vi "DequeueCmd.vi"(8 "error in (no error)":errorcluster, 11 "queue of text strings":refnum<queue>) -> (0 "error out":errorcluster, 1 "arguments":string[](array[string]), 2 "command":string="Default", 3 "queue (dup)":refnum<queue>)   [LabVIEW 2010]
doc: "This VI serves to dequeue a command from the string queue provided to the input. The queue sorts the command from the command line arguements, which can be included after the command. The arguements are separated by a colon (:) and will be output as a string array. The VI will also handle any error that exists in the error cluster by setting the command = Error with the error code and error string message as arguments.\n\nInputs:\nqueue - input queue (string)\nerror in - error input cluster\n\nOutputs:\ncommand - main state in the queue; this is used as the current state to be used by the case structure\narguments - command line arguments that were included with the command; separated by colon (:)\nqueue - duplicate reference for the queue\nerror out - error output cluster"
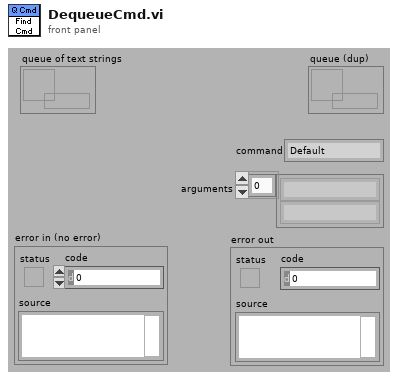
[diagram p1: front panel]
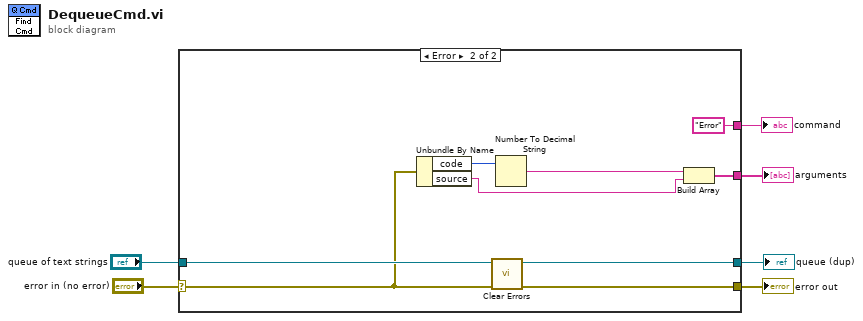
[diagram p0: block diagram]
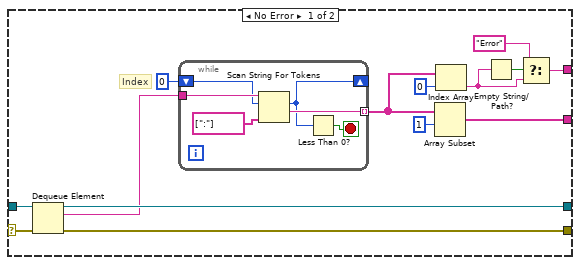
[diagram p2: hidden frame]
diagram:
  n1 = case shown="Error" "error in (no error)" {
    selector: "error in (no error)" -> [w8 w29]
    tunnel: [w20 w28] -> w6
    tunnel: "queue of text strings" -> [w18 w34]
    tunnel: [w17 w31] -> w4
    tunnel: [w13 w34] -> w3
    tunnel: [w12 "Error" ("token string")] -> w2
    frame No Error {
      # "Index"
      n2 = Dequeue Element(queue=w18, error in (no error)=w8) -> (queue out=w13:refnum<queue>, element=w7:string, error out=w20:errorcluster)  [unwired: 1 in, 1 out]
      n3 = while {
        tunnel: [w26] -> w15 mode=indexing
        tunnel: w7 -> [w24]
        shift-right: [w23] -> _
        shift-left: 0 ("offset past token") -> [w22]
        stop <- w25 stop-if-true
        n4 = Scan String For Tokens(6:string[] [":"] ("delimiters (\\s,\\t,\\r,\\n)"), 8:w22, 9:w24) -> (1:w26:string, 2:w23:i32)  [unwired: 3 in, 2 out]
        n5 = Less Than 0?(x=w23) -> (x < 0?=w25:bool)
      }
      n6 = Array Subset(array=w15, index=1) -> (w17:string[])  [unwired: 1 in]
      n7 = Index Array(array=w15, index=0) -> (element=w10:string)
      n8 = Empty String/Path?(string/path=w10) -> (empty?=w11:bool)
      n9 = Select(t="Error", s=w11, f=w10) -> (s? t:f=w12:string)
    }
    frame Error {
      n10 = Unbundle By Name(w29) -> ("code"=w32:i32, "source"=w27:string)
      n11 = call "Clear Errors.vi"("error in (no error)"=w29) -> ("error out"=w28:errorcluster)  [unwired: 6 in]
      n12 = Number To Decimal String(number=w32) -> (decimal integer string=w30:string)  [unwired: 1 in]
      n13 = Build Array(w30, w27) -> (w31:string[])
    }
  }
  "error out" <- w6
  "arguments" <- w4
  "command" <- w2
  "queue (dup)" <- w3
